vi "Acquire.vi"(8 "error in (no error)":errorcluster, 10 "Msg in":T1, 11 "FakePressureController in":refnum<class "Tapedrive_ESP301.lvclass">) -> (0 "error out":errorcluster, 1 "new command":string, 2 "Msg out":T1, 3 "FakePressureController out":refnum<class "Tapedrive_ESP301.lvclass">)   [LabVIEW 2011, in "Tapedrive_ESP301.lvclass"]
uses:
  Tapedrive_ESP301.lvclass
  DriverMsg.ctl
  OnOffTypeDef.ctl
  Tapedrive_ESP301.lvclass/Tapedrive_ESP301.ctl
  BaseDriver/BaseDriver.lvclass
  Newport ESP301.lvlib
panel:
  out "result":bool
  out "element":string
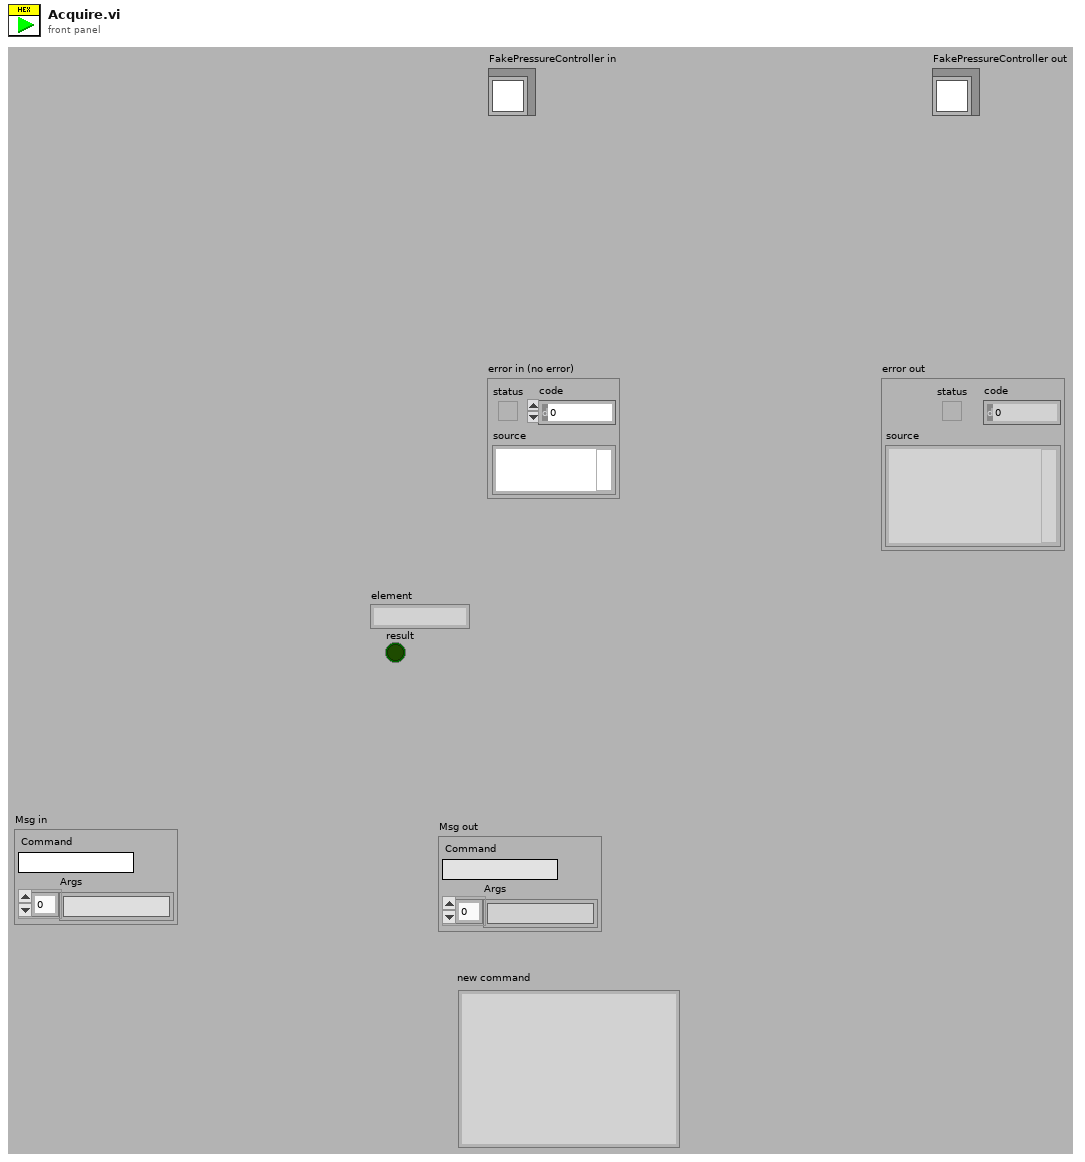
[diagram p1: front panel]
types:
  T1 = typedef "DriverMsg.ctl" = cluster{"Command":string, "Args":string[]}
  T2 = typedef "OnOffTypeDef.ctl" = enum16{"off", "on"}
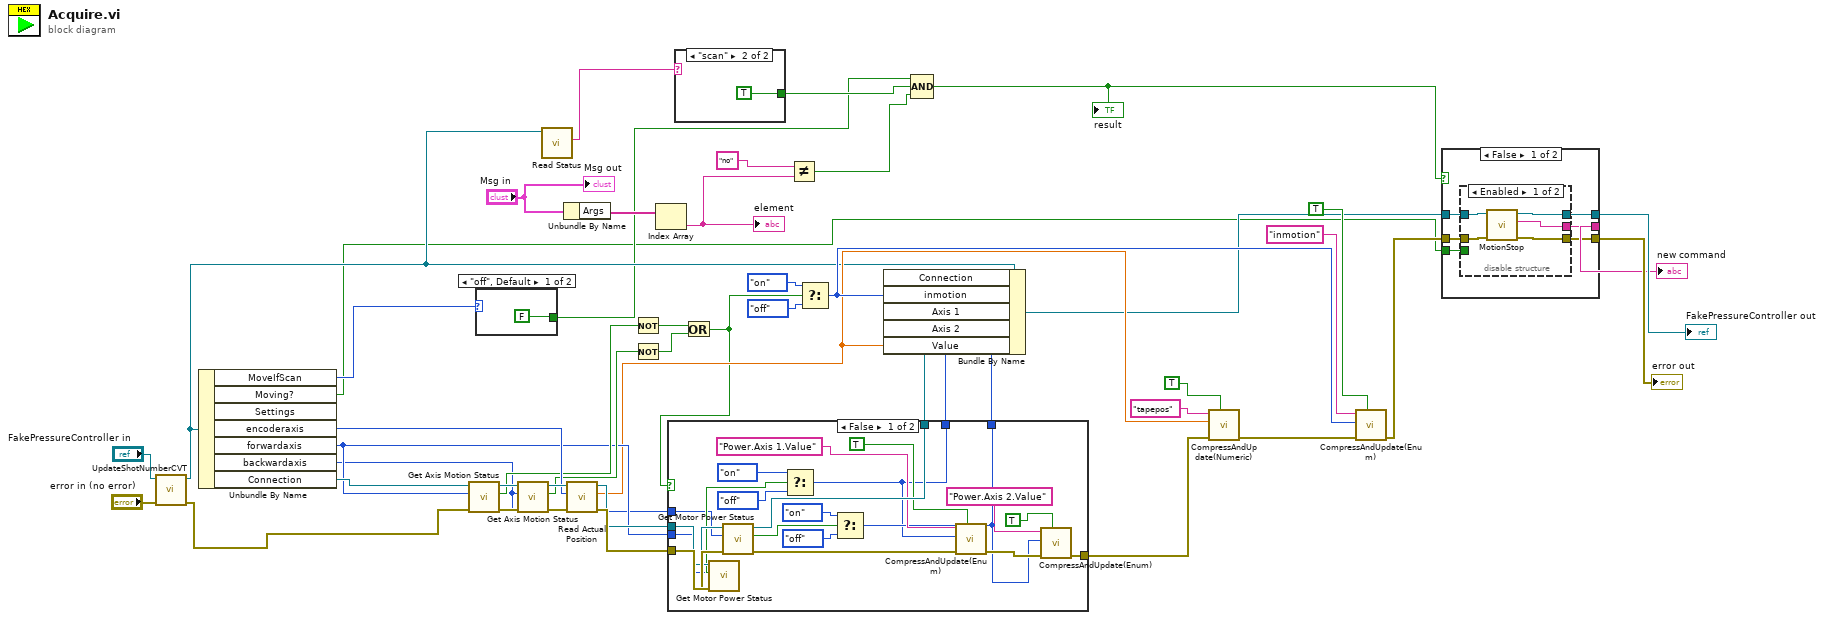
[diagram p0: block diagram]
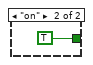
[diagram p2: hidden frame]
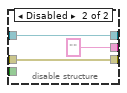
[diagram p3: hidden frame]
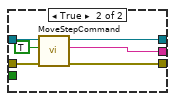
[diagram p4: hidden frame]
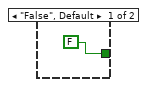
[diagram p5: hidden frame]
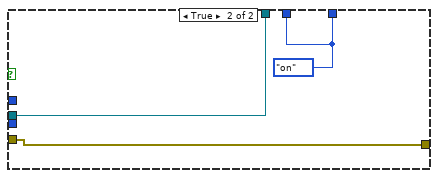
[diagram p6: hidden frame]
diagram:
  n1 = call "UpdateShotNumberCVT.vi"("error in (no error)"="error in (no error)", "BaseDriver in"="FakePressureController in") -> ("error out"=w2:errorcluster, "BaseDriver out"=w15:refnum<class "Tapedrive_ESP301.lvclass">)  [unwired: 8 in]
  n2 = Unbundle By Name(w15) -> ("MoveIfScan"=w6:T2, "Moving?"=w4:bool, "encoderaxis"=w40:i16, "forwardaxis"=w26:i16, "backwardaxis"=w25:i16, "Connection"=w44:refnum<visa-resource-name>)  [unwired: 1 out]
  n3 = call "Get Axis Motion Status.vi"("error in (no error)"=w2, "Axis (1)"=w26, "VISA resource name"=w44) -> ("error out"=w43:errorcluster, "Motion Done"=w38:bool, "VISA resource name out"=w42:refnum<visa-resource-name>)  [unwired: 2 in]
  n4 = case shown="\"off\", Default" w6 {
    tunnel: [FALSE ("force CVT update (false)") TRUE ("force CVT update (false)")] -> w5
    frame "off", Default {
    }
    frame "on" {
    }
  }
  n5 = call "Get Axis Motion Status.vi"("error in (no error)"=w43, "Axis (1)"=w25, "VISA resource name"=w42) -> ("error out"=w39:errorcluster, "Motion Done"=w37:bool, "VISA resource name out"=w41:refnum<visa-resource-name>)  [unwired: 2 in]
  n6 = call "Read Status.vi"("BaseDriver in"=w15) -> ("Status"=w14:string)  [unwired: 8 in, 2 out]
  n7 = Unbundle By Name("Msg in") -> ("Args"=w12:string[])
  n8 = call "Read Actual Position.vi"("error in (no error)"=w39, "Axis (1)"=w40, "VISA resource name"=w41) -> ("error out"=w29:errorcluster, "Position (units)"=w20:dbl, "VISA resource name out"=w28:refnum<visa-resource-name>)  [unwired: 2 in]
  n9 = Not(x=w38) -> (.not. x?=w35:bool)
  n10 = Not(x=w37) -> (.not. x?=w36:bool)
  n11 = Index Array(array=w12) -> (element=w11:string)  [unwired: 1 in]
  "element" <- w11
  n12 = case shown="\"scan\"" w14 {
    tunnel: [FALSE ("force CVT update (false)") TRUE ("force CVT update (false)")] -> w8
    frame "False", Default {
    }
    frame "scan" {
    }
  }
  n13 = Or(x=w35, y=w36) -> (x .or. y?=w1:bool)
  n14 = case shown="False" w1 {
    tunnel: w29 -> [w74 w75]
    tunnel: w28 -> [w72 w77]
    tunnel: [w70 w77] -> w27
    tunnel: w26 -> [w63 _]
    tunnel: w25 -> [w62 _]
    tunnel: [w55 w75] -> w24
    tunnel: [w54 w76] -> w22
    tunnel: [w53 w76] -> w21
    frame False {
      n15 = call "Get Motor Power Status.vi"("error in (no error)"=w74, "Axis (1)"=w63, "VISA resource name"=w72) -> ("error out"=w73:errorcluster, "Power Status"=w65:bool, "VISA resource name out"=w71:refnum<visa-resource-name>)  [unwired: 2 in]
      n16 = call "Get Motor Power Status.vi"("error in (no error)"=w73, "Axis (1)"=w62, "VISA resource name"=w71) -> ("error out"=w57:errorcluster, "Power Status"=w64:bool, "VISA resource name out"=w70:refnum<visa-resource-name>)  [unwired: 2 in]
      n17 = Select(t=OnOffTypeDef."on" ("Settings.inmotion"), s=w65, f=OnOffTypeDef."off" ("Settings.inmotion")) -> (s? t:f=w53:T2)
      n18 = Select(t=OnOffTypeDef."on" ("Settings.inmotion"), s=w64, f=OnOffTypeDef."off" ("Settings.inmotion")) -> (s? t:f=w54:T2)
      n19 = call "CompressAndUpdate(Enum).vi"("force CVT update (false)"=TRUE, "error in"=w57, "enum variant"=w53, "command or variable name"="Power.Axis 1.Value") -> ("error out"=w56:errorcluster)  [unwired: 7 in]
      n20 = call "CompressAndUpdate(Enum).vi"("force CVT update (false)"=TRUE, "error in"=w56, "enum variant"=w54, "command or variable name"="Power.Axis 2.Value") -> ("error out"=w55:errorcluster)  [unwired: 7 in]
    }
    frame True {
      w76 = OnOffTypeDef."on" ("Settings.inmotion")
    }
  }
  n21 = Not Equal?(x="no", y=w11) -> (x != y?=w9:bool)
  n22 = Select(t=OnOffTypeDef."on" ("Settings.inmotion"), s=w1, f=OnOffTypeDef."off" ("Settings.inmotion")) -> (s? t:f=w23:T2)
  n23 = Bundle By Name(cluster=w15, "Connection"=w27, "inmotion"=w23, "Axis 1"=w21, "Axis 2"=w22, "Value"=w20) -> (w19:refnum<class "Tapedrive_ESP301.lvclass">)
  n24 = Compound Arithmetic op=AND(w5, w8, w9) -> (w7:bool)
  "result" <- w7
  n25 = call "CompressAndUpdate(Numeric).vi"("force CVT update (false)"=TRUE, "error in"=w24, "Numeric"=w20, "command or variable name"="tapepos") -> ("error out"=w31:errorcluster)  [unwired: 7 in]
  n26 = call "CompressAndUpdate(Enum).vi"("force CVT update (false)"=TRUE, "error in"=w31, "enum variant"=w23, "command or variable name"="inmotion") -> ("error out"=w18:errorcluster)  [unwired: 7 in]
  n27 = case shown="False" w7 {
    tunnel: w19 -> [w83 w96]
    tunnel: w18 -> [w82 w94]
    tunnel: [w81 w93] -> w17
    tunnel: [w80 w95] -> w16
    tunnel: [w79 w97] -> w3
    tunnel: w4 -> [w78 _]
    frame False {
      n28 = disable-structure shown="Enabled" {
        disable-tunnel: w83 -> [w88 w90]
        disable-tunnel: w82 -> [w85 w89]
        disable-tunnel: [w86 w89] -> w81
        disable-tunnel: [w87 w90] -> w80
        disable-tunnel: [w84 "" ("new command")] -> w79
        disable-tunnel: w78 -> [_ _]
        frame Enabled {
          n29 = call "MotionStop.vi"("error in (no error)"=w85, "Tapedrive_ESP301 in"=w88) -> ("error out"=w86:errorcluster, "new command"=w84:string, "Tapedrive_ESP301 out"=w87:refnum<class "Tapedrive_ESP301.lvclass">)  [unwired: 7 in]
        }
        frame Disabled {
        }
      }
    }
    frame True {
      n30 = call "MoveStepCommand.vi"("error in (no error)"=w94, "MultiCVT"=TRUE, "Tapedrive_ESP301 in"=w96) -> ("error out"=w93:errorcluster, "String"=w97:string, "Tapedrive_ESP301.lvclass"=w95:refnum<class "Tapedrive_ESP301.lvclass">)  [unwired: 6 in]
    }
  }
  "error out" <- w17
  "FakePressureController out" <- w16
  "new command" <- w3
  "Msg out" <- "Msg in"
